vi "get sample header columns.vi"(0 "report file path":path=path "D:/Cascade/templates/Fields for Excel sheets.xlsx", 5 "Start Cell Name":string="a3", 7 "Stop Cell name":string="b22", 11 "error in (no error)":errorcluster) -> (1 "output cluster":cluster{"row":i32, "column":i32}, 2 "Worksheet Names":string[](array[string]), 3 "Headers w/o change":string[](array[string]), 4 "Column of Volume":i32, 6 "Columns":i32[](array[numeric]), 8 "Worksheet Names 2":string[](array[string]), 10 "row":i32, 13 "data":string[][](array[string]), 14 "Column Letters":string[](array[string]), 15 "error out":errorcluster)   [LabVIEW 2016]
uses:
  <vilib>/addons/_office/excel.llb/Excel Get Data ([str]).vi
  <vilib>/Utility/NIReport.llb/NI_report.lvclass
  <vilib>/addons/_office/NI_ReportGenerationToolkit.lvlib
  <vilib>/Utility/NIReport.llb/Excel/NI_Excel.lvclass
panel:
  in  "Header Rows to remove":i32
  out "column max value":i32
  out "row max value":i32
  out "start of last occupied row":string
  out "last occupied cell's name":string
  out "size(s)":i32[](array[numeric])
  out "column":i32
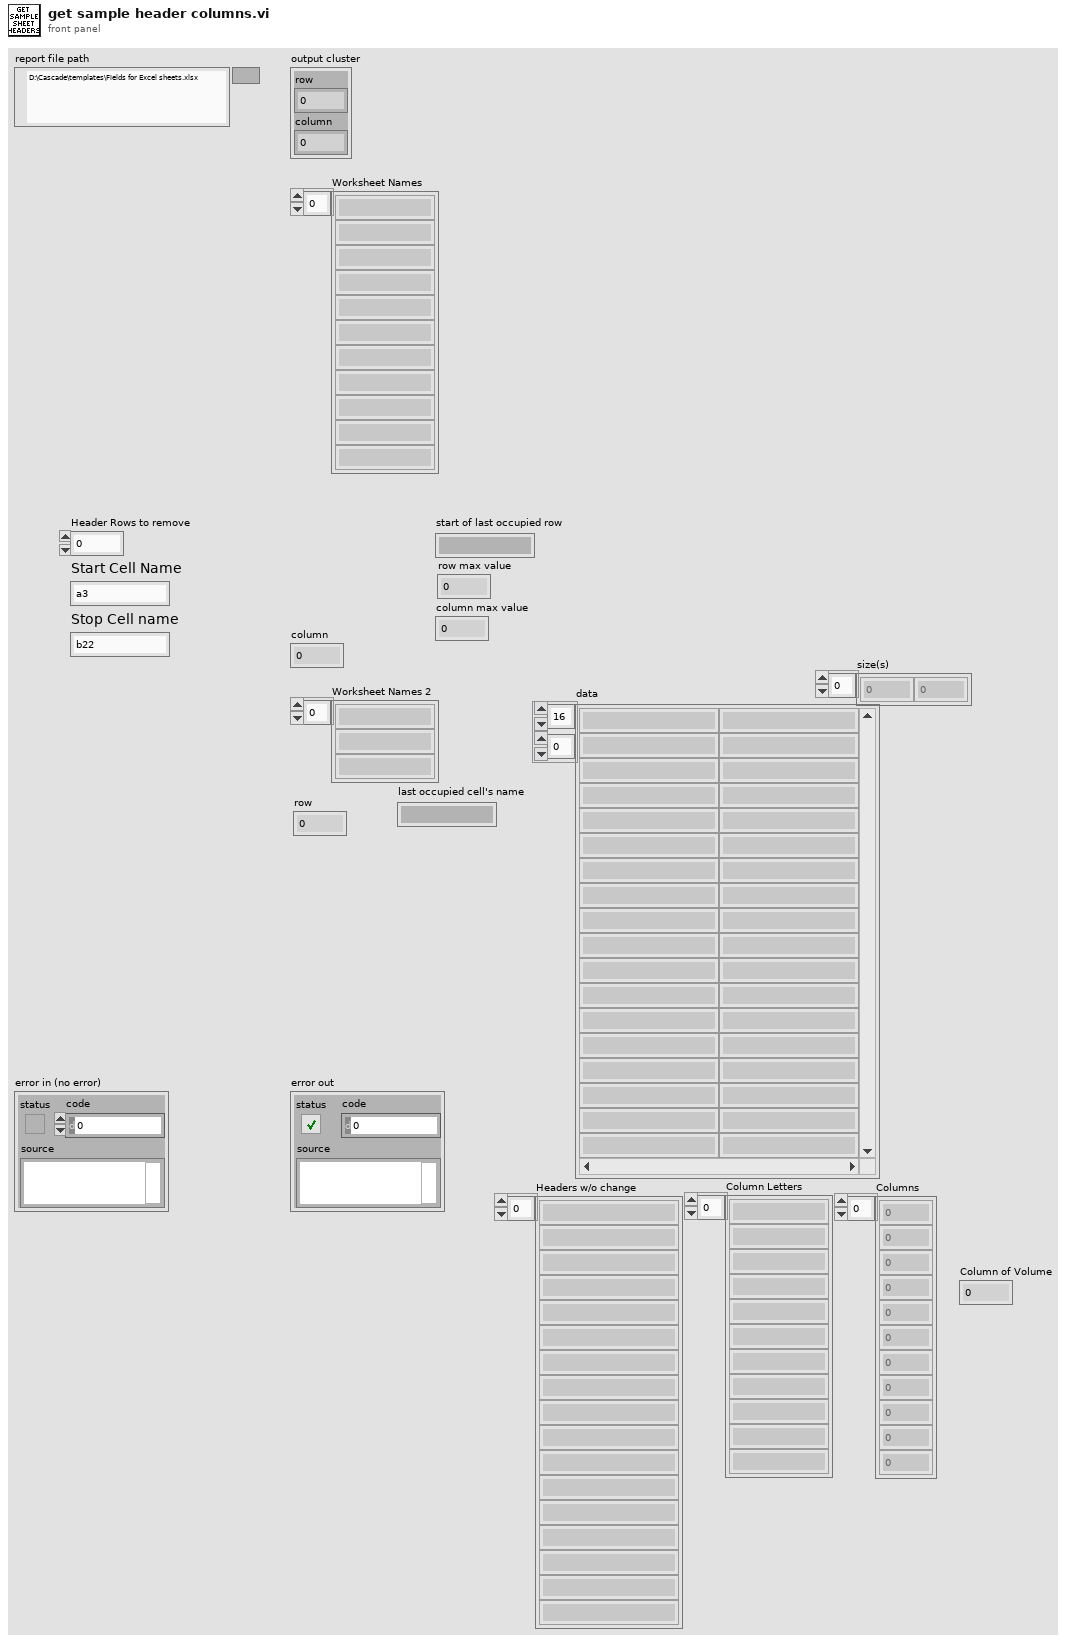
[diagram p1: front panel]
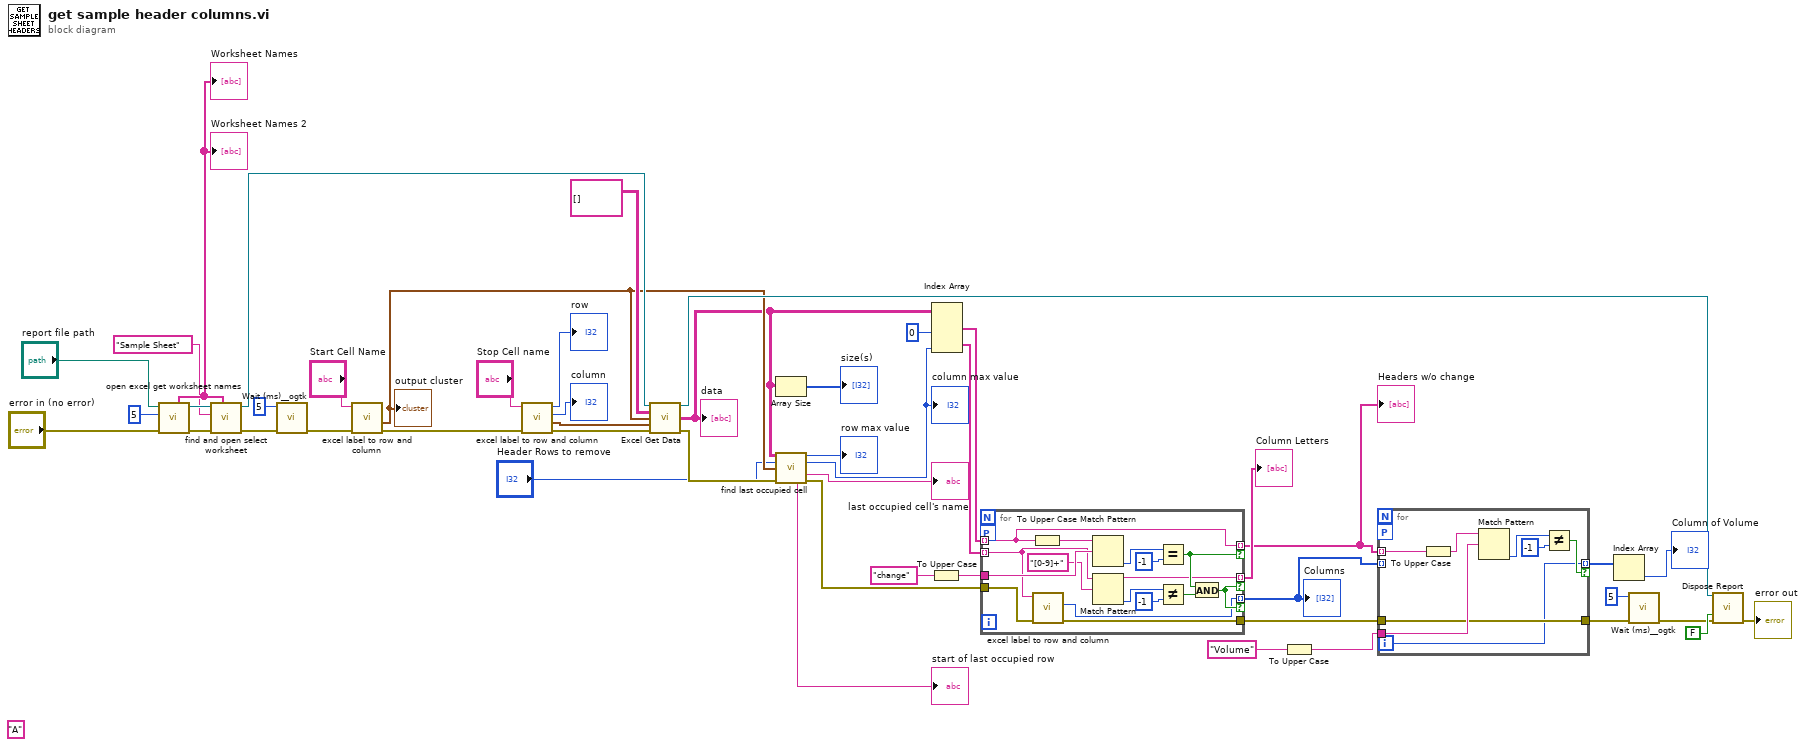
[diagram p0: block diagram]
diagram:
  (unwired) "A"
  n1 = call "open excel get worksheet names.vi"("error in (no error)"="error in (no error)", "milliseconds to wait"=u32 5, "report file path"="report file path") -> ("error out"=w45:errorcluster, "NI_report out"=w46:refnum<class "NI_report.lvclass">, "Worksheet Names"=w47:string[])  [unwired: 3 in, 3 out]
  "Worksheet Names" <- w47
  "Worksheet Names 2" <- w47
  n2 = call "find and open select worksheet.vi"("Worksheet Names"=w47, "error in (no error)"=w45, "Worksheet Name in"="Sample Sheet" ("Worksheet Name 1"), "NI_report in"=w46) -> ("error out"=w33:errorcluster, "NI_report out"=w36:refnum<class "NI_report.lvclass">)  [unwired: 5 in, 1 out]
  n3 = call <userlib>:"Wait (ms)__ogtk.vi"("error in (no error)"=w33, "milliseconds to wait"=u32 5) -> ("error out"=w39:errorcluster)  [unwired: 8 in, 1 out]
  n4 = call "excel label to row and column.vi"("error in (no error)"=w39, "cell's name"="Start Cell Name") -> ("error IO"=w40:errorcluster, "output cluster"=w21:cluster{"row":i32, "column":i32})  [unwired: 5 in, 3 out]
  "output cluster" <- w21
  n5 = call "excel label to row and column.vi"("error in (no error)"=w40, "cell's name"="Stop Cell name") -> ("error IO"=w42:errorcluster, "output cluster"=w41:cluster{"row":i32, "column":i32}, "column"=→"column":i32, "row"=→"row":i32)  [unwired: 5 in, 1 out]
  n6 = call-poly <vilib>:"Excel Get Data.vi"("report in"=w36, "data type"=string[][] [] ("Worksheet Names 2"), "start (-1, -1)"=w21, "end (-1, -1)"=w41, "error in (no error)"=w42) -> ("report out"=w25:refnum<class "NI_report.lvclass">, "data"=w17:string[][], "error out"=w23:errorcluster)  [unwired: 8 in]
  "data" <- w17
  n7 = Array Size(array=w17) -> (size(s)=→"size(s)":i32[])
  n8 = call "find last occupied cell.vi"("data"=w17, "Header Rows to remove"="Header Rows to remove", "sub array start"=w21, "error in (no error)"=w23) -> ("row max value"=→"row max value":i32, "column max value"=w13:i32, "last occupied cell's name"=→"last occupied cell's name":string, "start of last occupied row"=→"start of last occupied row":string, "error out"=w14:errorcluster)  [unwired: 5 in, 2 out]
  "column max value" <- w13
  n9 = To Upper Case(1:"change" ("regular expression")) -> (0:w15:string)
  n10 = Index Array(array=w17, index (col) #1=0 ("index (col)"), index (col) #2=w13) -> (element #1=w10:string[], element #2=w11:string[])  [unwired: 2 in]
  n11 = for {
    tunnel: w11 -> [w55] mode=indexing
    tunnel: [w59] -> w6 mode=indexing if=w52
    tunnel: w15 -> [w64]
    tunnel: [w49] -> w1 mode=indexing if=w61
    tunnel: w10 -> [w49] mode=indexing
    tunnel: w14 -> [w54]
    tunnel: [w53] -> w7
    tunnel: [w51] -> w5 mode=indexing if=w52
    workers-P: _ -> [_]
    n12 = To Upper Case(1:w49) -> (0:w50:string)
    n13 = call "excel label to row and column.vi"("error in (no error)"=w54, "cell's name"=w55) -> ("error IO"=w53:errorcluster, "column"=w51:i32)  [unwired: 5 in, 3 out]
    n14 = Match Pattern(string=w50, regular expression=w64) -> (offset past match=w63:i32)  [unwired: 1 in, 3 out]
    n15 = Match Pattern(string=w55, regular expression="[0-9]+") -> (before substring=w59:string, offset past match=w57:i32)  [unwired: 1 in, 2 out]
    n16 = Equal?(x=w63, y=-1) -> (x = y?=w61:bool)
    n17 = Not Equal?(x=w57, y=-1) -> (x != y?=w56:bool)
    n18 = And(x=w61, y=w56) -> (x .and. y?=w52:bool)
  }
  "Headers w/o change" <- w1
  "Column Letters" <- w6
  "Columns" <- w5
  n19 = To Upper Case(1:"Volume" ("regular expression")) -> (0:w8:string)
  n20 = for {
    tunnel: w1 -> [w68] mode=indexing
    tunnel: w7 -> [w67]
    tunnel: w8 -> [w70]
    tunnel: [w67] -> w2
    tunnel: [w65] -> w4 mode=indexing if=w66
    tunnel: w5 -> [_] mode=indexing
    workers-P: _ -> [_]
    i -> [w65]
    n21 = To Upper Case(1:w68) -> (0:w69:string)
    n22 = Match Pattern(string=w69, regular expression=w70) -> (offset past match=w71:i32)  [unwired: 1 in, 3 out]
    n23 = Not Equal?(x=w71, y=-1) -> (x != y?=w66:bool)
  }
  n24 = Index Array(array=w4) -> (element=→"Column of Volume":i32)  [unwired: 1 in]
  n25 = call <userlib>:"Wait (ms)__ogtk.vi"("error in (no error)"=w2, "milliseconds to wait"=u32 5) -> ("error out"=w28:errorcluster)  [unwired: 8 in, 1 out]
  n26 = call-dynamic "Dispose Report.vi"("report in"=w25, "save changes? (F)"=FALSE, "error in (no error)"=w28) -> ("error out"=→"error out":errorcluster)  [unwired: 12 in]
